vi "update_time.vi"(11 "Event in":refnum<class "NISAST Event.lvclass">) -> ()   [LabVIEW 2021, in "Clock.xctl"]
uses:
  Clock.xctl
  <resource>/importtools/Common/Event/NISAST Event.lvclass
  message.ctl
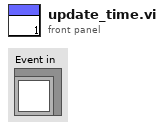
[diagram p1: front panel]
types:
  T1 = typedef "Clock.xctl/message.ctl" = cluster{"hour":refnum<vi>, "minute":refnum<vi>, "second":refnum<vi>}
  T2 = typedef "NISAST Event.lvclass/Event Registeration Refnum.ctl" = refnum<event-registration>
  T3 = typedef "LVDateTimeRec.ctl" = cluster{"fractional second":dbl, "second":i32, "minute":i32, "hour":i32, "day of month":i32, "month":i32, "year":i32, "day of week":i32, "day of year":i32, "DST":i32}
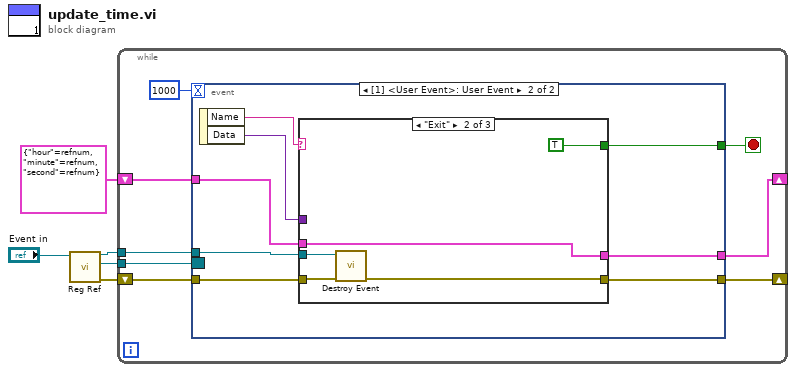
[diagram p0: block diagram]
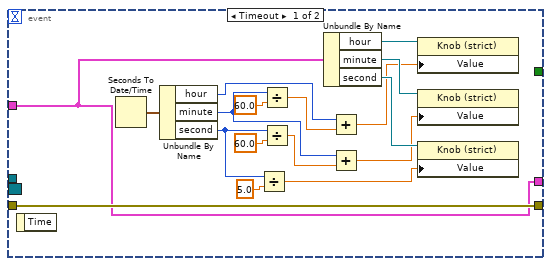
[diagram p2: hidden frame]
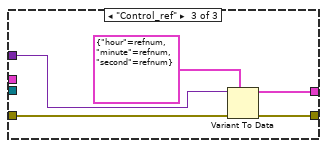
[diagram p4: hidden frame]
diagram:
  n1 = call-dynamic "Reg Ref.vi"("Event in"="Event in") -> ("error out"=w2:errorcluster, "Event Registration Refnum"=w5:T2, "Event out"=w1:refnum<class "NISAST Event.lvclass">)  [unwired: 8 in]
  n2 = while {
    tunnel: w5 -> [w12]
    shift-right: [w11] -> _
    shift-left: T1 {"hour"=refnum, "minute"=refnum, "second"=refnum} ("message") -> [w10]
    shift-right: [w8] -> _
    shift-left: w2 -> [w9]
    tunnel: w1 -> [w6]
    stop <- w7 stop-if-true
    n3 = event shown="[1] <User Event>: User Event" {
      selector: w12 -> [_ _]
      dyn-events: _ -> [_ _]
      timeout: 1000 -> [_ _]
      tunnel: [w14 w36] -> w11
      tunnel: w10 -> [w14 w35]
      tunnel: w9 -> [w15 w34]
      tunnel: [w15 w33] -> w8
      tunnel: [_ w32] -> w7
      tunnel: w6 -> [_ w31]
      event Timeout {
        n4 = event-data() -> ()  [unwired: 1 in, 1 out]
        n5 = Seconds To Date/Time() -> (date time rec=w30:T3)  [unwired: 2 in]
        n6 = Unbundle By Name(w30) -> ("hour"=w25:i32, "minute"=w20:i32, "second"=w17:i32)
        n7 = Divide(x=w17, y=5.0) -> (x/y=w16:dbl)
        n8 = Divide(x=w20, y=60.0) -> (x/y=w24:dbl)
        n9 = Divide(x=w17, y=60.0) -> (x/y=w21:dbl)
        n10 = Unbundle By Name(w14) -> ("hour"=w27:refnum<vi>, "minute"=w28:refnum<vi>, "second"=w29:refnum<vi>)
        n11 = Add(x=w25, y=w24) -> (x+y=w23:dbl)
        n12 = Add(x=w20, y=w21) -> (x+y=w19:dbl)
        n13 = property class="Knob (strict)"(reference=w27, "Value"=w23) -> ()  [unwired: 1 in, 2 out]
        n14 = property class="Knob (strict)"(reference=w28, "Value"=w19) -> ()  [unwired: 1 in, 2 out]
        n15 = property class="Knob (strict)"(reference=w29, "Value"=w16) -> ()  [unwired: 1 in, 2 out]
      }
      event User Event {
        n16 = event-data() -> ("Name"=w38:string, "Data"=w37:variant)  [unwired: 1 in]
        n17 = case shown="\"Exit\"" w38 {
          tunnel: w37 -> [_ _ w49]
          tunnel: [w40 w45 w46] -> w36
          tunnel: w35 -> [w40 w45 _]
          tunnel: w34 -> [w39 w43 w48]
          tunnel: [w39 w41 w47] -> w33
          tunnel: [_ TRUE _] -> w32
          tunnel: w31 -> [_ w42 _]
          frame Default {
          }
          frame "Exit" {
            n18 = call-dynamic "Destroy Event.vi"("error in (no error)"=w43, "Event in"=w42) -> ("error out"=w41:errorcluster)  [unwired: 8 in, 1 out]
          }
          frame "Control_ref" {
            n19 = Variant To Data(error in=w48, type=T1 {"hour"=refnum, "minute"=refnum, "second"=refnum} ("message"), Variant=w49) -> (data=w46:T1, error out=w47:errorcluster)
          }
        }
      }
    }
  }
